vi "Stop Task.vi"(8 "error in":errorcluster, 11 "NI Digital Input in":refnum<class "NI Digital Input.lvclass">) -> (0 "error out":errorcluster, 3 "NI Digital Input out":refnum<class "NI Digital Input.lvclass">)   [LabVIEW 2023, in "HardwareAbstractionLayer_LVOOP.lvlib" / "NI Digital Input.lvclass"]
uses:
  NI Digital Input.lvclass
  NI Digital Input.lvclass/NI Digital Input.ctl
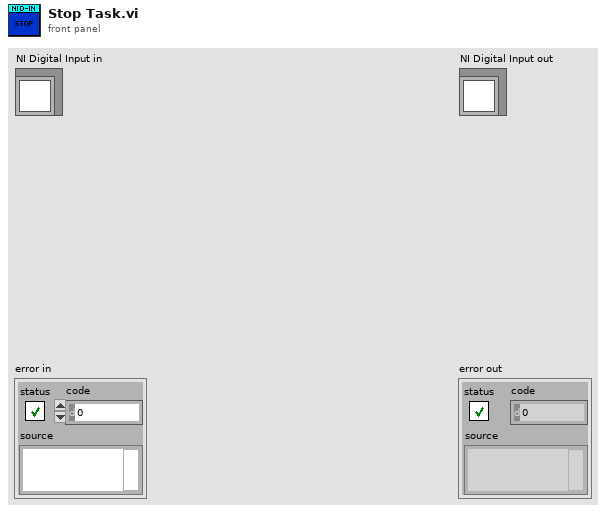
[diagram p1: front panel]
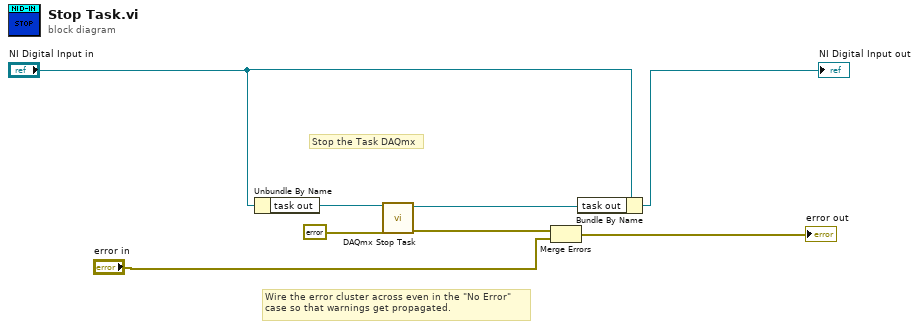
[diagram p0: block diagram]
diagram:
  # "Stop the Task DAQmx"
  # "Wire the error cluster across even in the \"No Error\"\ncase so that warnings get propagated."
  n1 = Unbundle By Name("NI Digital Input in") -> ("task out"=w5:refnum<k21>)
  n2 = call <vilib>:"DAQmx Stop Task.vi"("task/channels in"=w5, "error in"=errorcluster {"status"=FALSE, "code"=0, "source"=""}) -> ("task out"=w4:refnum<k21>, "error out"=w8:errorcluster)  [unwired: 12 in]
  n3 = Merge Errors(w8, "error in") -> (→"error out":errorcluster)
  n4 = Bundle By Name(cluster="NI Digital Input in", "task out"=w4) -> (→"NI Digital Input out":refnum<class "NI Digital Input.lvclass">)
